vi "Parse-Filter_Scanned_Indices.vi"(9 "Existing Indices":T3[](array[typedef]), 11 "Potential New Walls":T1[](array[typedef])) -> (1 "Existing Indices Out":T3[](array[typedef]), 3 "New Wall Indices":i32[](array[numeric]))   [LabVIEW 2020]
doc: "<B>Description:</B> Takes an array of barrier indices and for each one, checks if absolute difference between it and every Existing Index is greater than the grace band. If it is, it is a new index and is added to the Existing indexes as such. Otherwise, it is ignored.\n\n<B>Date:</B> 03/2019\n<B>Author:</B> Luke Jarocki, Choose Movement Consulting, LLC"
uses:
  Controls/Scan_Values.ctl
  Controls/Wall Data.ctl
  Controls/TileColor.ctl
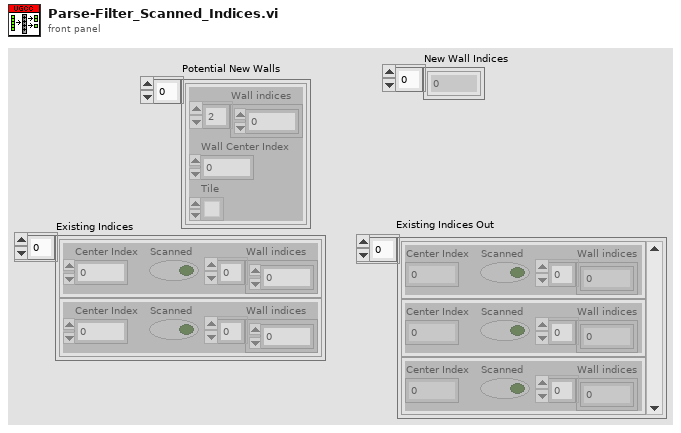
[diagram p1: front panel]
types:
  T1 = typedef "Wall Data.ctl" = cluster{"Wall indices":i32[], "Wall Center Index":i32, "Tile":T2}
  T2 = typedef "TileColor.ctl" = u16
  T3 = typedef "Scan_Values.ctl" = cluster{"Center Index":i32, "Scanned":bool, "Wall indices":i32[]}
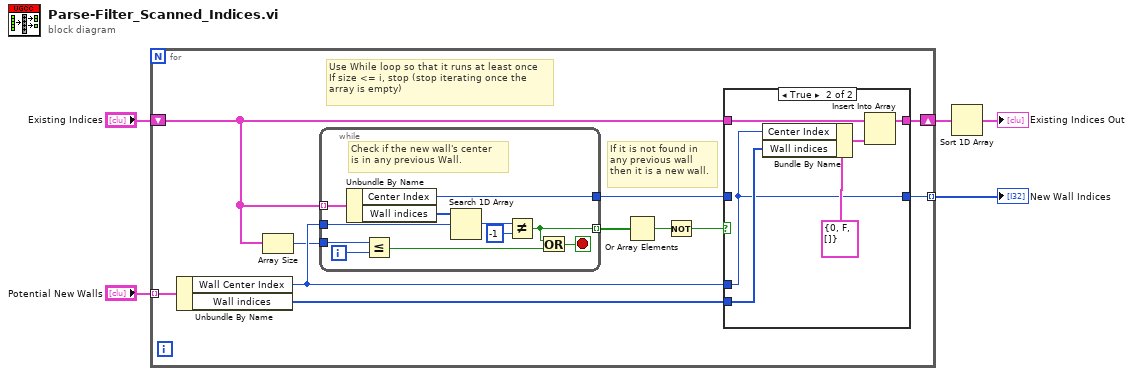
[diagram p0: block diagram]
diagram:
  n1 = for {
    shift-right: [w16] -> w4
    shift-left: "Existing Indices" -> [w7]
    tunnel: "Potential New Walls" -> [w15] mode=indexing
    tunnel: [w11] -> w1 mode=indexing
    # "Use While loop so that it runs at least once\nIf size <= i, stop (stop iterating once the\narray is empty)"
    # "If it is not found in\nany previous wall\nthen it is a new wall."
    n2 = Unbundle By Name(w15) -> ("Wall Center Index"=w14:i32, "Wall indices"=w13:i32[])
    n3 = Array Size(array=w7) -> (size(s)=w6:i32)
    n4 = while {
      tunnel: w7 -> [w27] mode=indexing
      tunnel: w14 -> [w25]
      tunnel: [w19] -> w10 mode=indexing
      tunnel: [w22] -> w12
      tunnel: w6 -> [w21]
      i -> [w20]
      stop <- w18 stop-if-true
      # "Check if the new wall's center\nis in any previous Wall."
      n5 = Unbundle By Name(w27) -> ("Center Index"=w22:i32, "Wall indices"=w26:i32[])
      n6 = Less Or Equal?(x=w21, y=w20) -> (x <= y?=w17:bool)
      n7 = Search 1D Array(1D array=w26, element=w25) -> (index of element=w24:i32)  [unwired: 1 in]
      n8 = Not Equal?(x=w24, y=-1) -> (x != y?=w19:bool)
      n9 = Or(x=w19, y=w17) -> (x .or. y?=w18:bool)
    }
    n10 = Or Array Elements(Boolean array=w10) -> (logical OR=w9:bool)
    n11 = Not(x=w9) -> (.not. x?=w8:bool)
    n12 = case shown="True" w8 {
      tunnel: w7 -> [w29 w35]
      tunnel: [w29 w34] -> w16
      tunnel: w14 -> [_ w30]
      tunnel: w13 -> [_ w31]
      tunnel: w12 -> [w28 _]
      tunnel: [w28 w30] -> w11
      frame False {
      }
      frame True {
        n13 = Bundle By Name(cluster=T3 {"Center Index"=0, "Scanned"=FALSE, "Wall indices"=[]} ("new element/subarray"), "Center Index"=w30, "Wall indices"=w31) -> (w32:T3)
        n14 = Insert Into Array(array=w35, new element=w32) -> (w34:T3[])  [unwired: 1 in]
      }
    }
  }
  "New Wall Indices" <- w1
  n15 = Sort 1D Array(array=w4) -> (sorted array=→"Existing Indices Out":T3[])
